vi "Validate Time Differences.vi"(6 "maximum deviation":dbl=0.001, 8 "error in (no error)":errorcluster, 9 "expected value":dbl, 10 "time differences":dbl[](array[numeric]), 11 "CAN Loopback Tests in":refnum<class "CAN Loopback Tests.lvclass">) -> (0 "error out":errorcluster, 3 "CAN Loopback Tests out":refnum<class "CAN Loopback Tests.lvclass">)   [LabVIEW 2017, in "CAN Loopback Tests.lvclass"]
uses:
  CAN Loopback Tests.lvclass
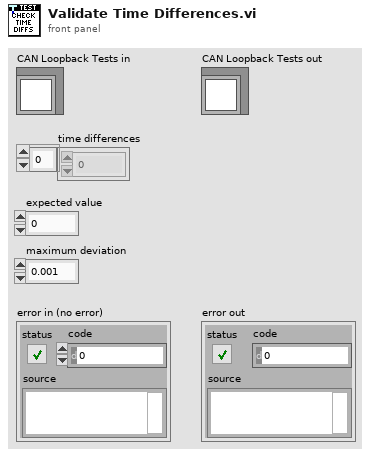
[diagram p1: front panel]
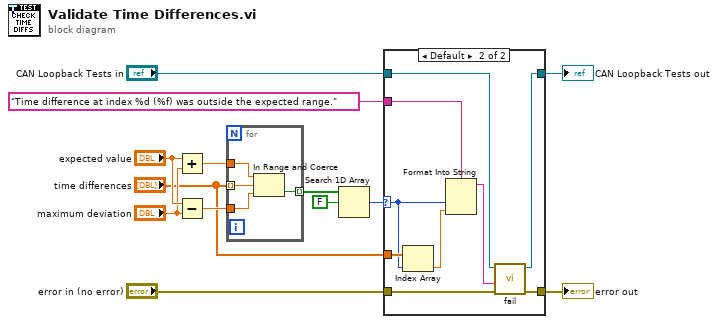
[diagram p0: block diagram]
diagram:
  n1 = Add(x="expected value", y="maximum deviation") -> (x+y=w5:dbl)
  n2 = Subtract(x="expected value", y="maximum deviation") -> (x-y=w6:dbl)
  n3 = for {
    tunnel: "time differences" -> [w17] mode=indexing
    tunnel: w6 -> [w16]
    tunnel: w5 -> [w15]
    tunnel: [w14] -> w3 mode=indexing
    n4 = In Range and Coerce(upper limit=w15, x=w17, lower limit=w16) -> (In Range?=w14:bool)  [unwired: 1 out]
  }
  n5 = Search 1D Array(1D array=w3, element=FALSE) -> (index of element=w2:i32)  [unwired: 1 in]
  n6 = case shown="Default" w2 {
    selector: w2 -> [_ w20]
    tunnel: "error in (no error)" -> [w18 w28]
    tunnel: [w18 w27] -> w12
    tunnel: "CAN Loopback Tests in" -> [w19 w26]
    tunnel: [w19 w25] -> w10
    tunnel: "Time difference at index %d (%f) was outside the expected range." ("format string") -> [_ w23]
    tunnel: "time differences" -> [_ w22]
    frame -1 {
    }
    frame Default {
      n7 = Index Array(array=w22, index=w20) -> (element=w21:dbl)
      n8 = Format Into String(format string=w23, w20, w21) -> (resulting string=w24:string)  [unwired: 2 in, 1 out]
      n9 = call-dynamic "fail.vi"("error in (no error)"=w28, "message (\"\")"=w24, "TestCase in"=w26) -> ("error out"=w27:errorcluster, "TestCase out"=w25:refnum<class "CAN Loopback Tests.lvclass">)  [unwired: 7 in]
    }
  }
  "CAN Loopback Tests out" <- w10
  "error out" <- w12
